vi "Z900_navX_Util_DecodeProtocol_Int32.vi"(1 "Little Endian":u8[](array[numeric])) -> (0 "Int32":i32[](array[numeric]))   [LabVIEW 2015, in "navX Library v2.lvlib"]
uses:
  navX Library v2.lvlib
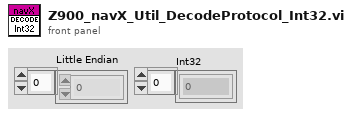
[diagram p1: front panel]
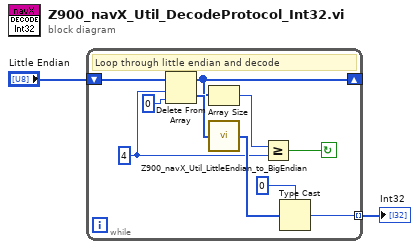
[diagram p0: block diagram]
diagram:
  n1 = while {
    shift-right: [w6] -> _
    shift-left: "Little Endian" -> [w12]
    tunnel: [w7] -> w1 mode=indexing
    stop <- w3 continue-if-true
    w4 = 4 ("length")
    # "Loop through little endian and decode"
    n2 = Delete From Array(array=w12, length=w4, index=0) -> (deleted portion=w8:u8[], array with subset deleted=w6:u8[])
    n3 = Array Size(array=w6) -> (size(s)=w5:i32)
    n4 = call "Z900_navX_Util_LittleEndian_to_BigEndian.vi"("Little Endian"=w8) -> ("Big Endian"=w10:u8[])
    n5 = Greater Or Equal?(x=w5, y=w4) -> (x >= y?=w3:bool)
    n6 = Type Cast(type=0, x=w10) -> (*(type *) &x=w7:i32)
  }
  "Int32" <- w1
